vi "Map Collection - Comparing Test Results.vi"() -> ()   [LabVIEW 2023]
doc: "This VI demonstrates basic use of the map data type. Maps are used to create a collection of keys and associate each unique key with a value. The user selects the two data types used for the keys and for the values.\n\nThis example uses maps to comparing actual test measurements of drinking water against a list of allowed contaminant levels and showing any result that is above accepted levels."
panel:
  out "actual levels":map{string, dbl[unit]}(c390)
  out "maximum levels":map{string, dbl[unit]}(c390)
  out "unsafe levels":map{string, dbl[unit]}(c390)
  # "Overview: This VI demonstrates basic use of the map data type. Maps are used to create a collection of keys and associate each unique key with a value. The user selects the two data types used for the keys and for the values.\n\nThis example uses maps to comparing actual test measurements of drinking water against a list of allowed contaminant levels and showing any result that is above accepted levels.\n\nInstructions:\n1. Run the VI. \n2. Observe that the unsafe levels lists all of the entries in the actual levels that are either above the maximum levels or not listed in maximum levels.\n3. Open the block diagram and review further commentary there."
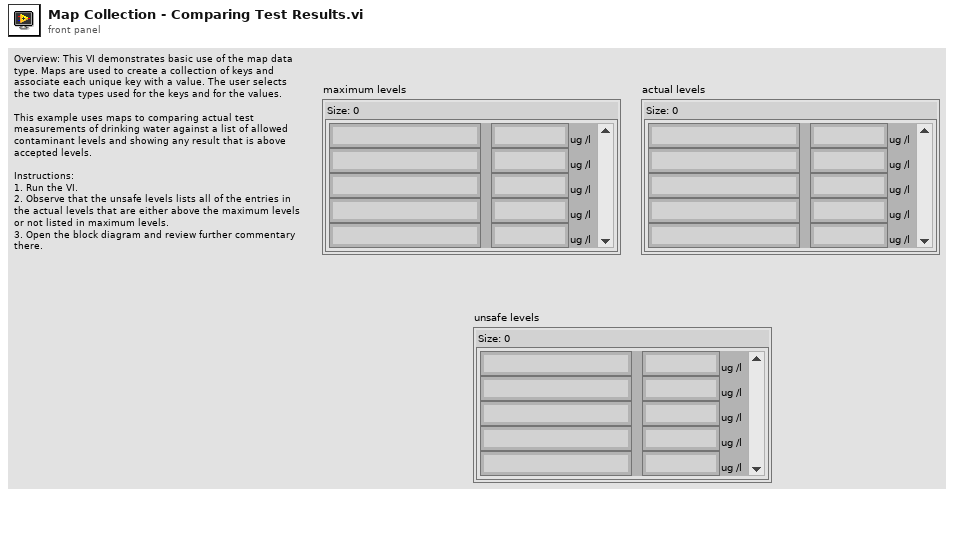
[diagram p1: front panel]
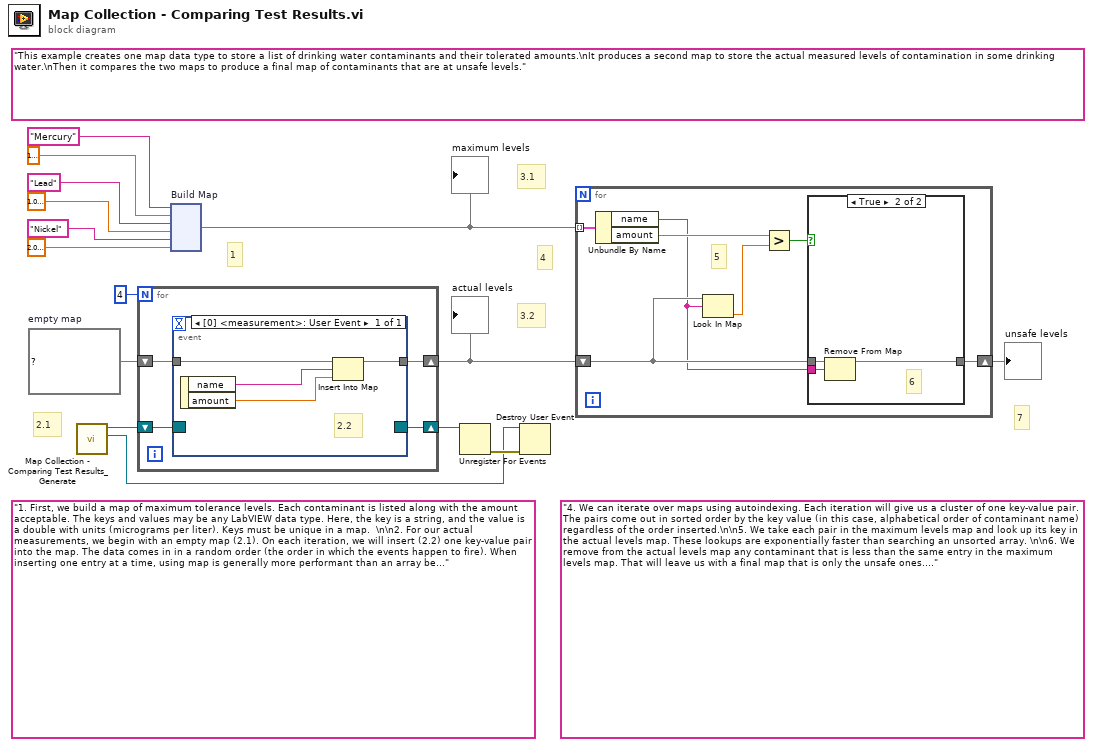
[diagram p0: block diagram]
diagram:
  (unwired) "This example creates one map data type to store a list of drinking water contaminants and their tolerated amounts.\nIt produces a second map to store the actual measured levels of contamination in some drinking water.\nThen it compares the two maps to produce a final map of contaminants that are at unsafe levels." ("L10n_heading")
  w1 = map{string, dbl[unit]} {}  # empty map
  (unwired) "4. We can iterate over maps using autoindexing. Each iteration will give us a cluster of one key-value pair. The pairs come out in sorted order by the key value (in this case, alphabetical order of contaminant name) regardless of the order inserted.\n\n5. We take each pair in the maximum levels map and look up its key in the actual levels map. These lookups are exponentially faster than searching an unsorted array. \n\n6. We remove from the actual levels map any contaminant that is less than the same entry in the maximum levels map. That will leave us with a final map that is only the unsafe ones.\n\n7. Finally, we display the results. Any contaminant that wasn't in our maximum levels map at all (Benzene) is included in the unsafe levels map.\n\nFor more advanced use of the map, please see:\nexamples\\Design Patterns\\Registration Map\\Registration Map Usage.lvproj" ("L10n_right")
  (unwired) "1. First, we build a map of maximum tolerance levels. Each contaminant is listed along with the amount acceptable. The keys and values may be any LabVIEW data type. Here, the key is a string, and the value is a double with units (micrograms per liter). Keys must be unique in a map.  \n\n2. For our actual measurements, we begin with an empty map (2.1). On each iteration, we will insert (2.2) one key-value pair into the map. The data comes in in a random order (the order in which the events happen to fire). When inserting one entry at a time, using map is generally more performant than an array because of the way data is stored in memory. Arrays are optimized for operations on the whole block of data; maps are optimized for per-entry operations.\n\n3. Notice that although the items were added to the two maps in different orders, they are both (3.1, 3.2) displayed sorted by key (name). Maps always store their items in sorted order so displaying ordered information requires no extra performance overhead." ("L10n_left")
  # "3.2"
  # "3.1"
  # "4"
  # "7"
  # "2.1"
  # "1"
  n1 = call "Map Collection - Comparing Test Results_Generate.vi"() -> ("measurement event refnum"=w5:refnum<user-event>, "registration refnum"=w8:refnum<event-registration>)  [unwired: 10 in]
  n2 = for {
    N: 4 -> [_]
    shift-right: [w17] -> w2
    shift-left: w1 -> [w18]
    shift-right: [w16] -> w7
    shift-left: w8 -> [w19]
    n3 = event shown="[0] <measurement>: User Event" {
      selector: w19 -> [_]
      dyn-events: [_] -> w16
      timeout: _ -> [_]
      tunnel: w18 -> [w23]
      tunnel: [w22] -> w17
      event User Event {
        # "2.2"
        n4 = event-data() -> ("name"=w21:string, "amount"=w20:dbl[unit])  [unwired: 1 in]
        n5 = Insert Into Map(map in=w23, key=w21, value=w20) -> (map out=w22:map{string, dbl[unit]})  [unwired: 2 out]
      }
    }
  }
  "actual levels" <- w2
  n6 = node "Build Map"("Mercury" ("name"), dbl[unit] 1e-06 ("amount"), "Lead" ("name"), dbl[unit] 1.0000000000000003e-05 ("amount"), "Nickel" ("name"), dbl[unit] 2.0000000000000005e-05 ("amount")) -> (w3:map{string, dbl[unit]})
  "maximum levels" <- w3
  n7 = Unregister For Events(event registration refnum=w7) -> (error out=w6:errorcluster)  [unwired: 1 in]
  n8 = Destroy User Event(user event=w5, error in=w6) -> ()  [unwired: 1 out]
  n9 = for {
    tunnel: w3 -> [w30] mode=indexing
    shift-right: [w24] -> w4
    shift-left: w2 -> [w26]
    # "5"
    n10 = Unbundle By Name(w30) -> ("name"=w25:string, "amount"=w29:dbl[unit])
    n11 = Look In Map(map=w26, key=w25) -> (value=w28:dbl[unit])  [unwired: 1 in, 1 out]
    n12 = Greater?(x=w29, y=w28) -> (0:w27:bool)
    n13 = case shown="True" w27 {
      tunnel: w26 -> [w31 w34]
      tunnel: w25 -> [_ w33]
      tunnel: [w31 w32] -> w24
      frame False {
      }
      frame True {
        # "6"
        n14 = Remove From Map(10:w33, 11:w34) -> (3:w32:map{string, dbl[unit]})  [unwired: 2 out]
      }
    }
  }
  "unsafe levels" <- w4
